vi "Load-GUI-values-from-file.vi"(8 "error in":errorcluster, 10 "UI ref. in":refnum<data-value>, 11 "Data ref. in":refnum<data-value>) -> (0 "error IO":errorcluster, 2 "UI ref.":refnum<data-value>, 3 "Data ref.":refnum<data-value>)   [LabVIEW 2013, in "CameraVision.lvlib" / "CV-Main.lvclass"]
doc: "This function loads and overwrites new values for the GUI parameters. The values are obtained from an .xml settings file. The user is warned that the parameters will be overwritten and has the possibility to cancel the operation.\nDepending on the 'Settings source' GUI control, 4 cases are possible:\n- 'Custom': the 'Load settings' button is disabled, no action is taken.\n- 'Default': the default values of the GUI parameters are loaded from '<Application>\\Program data\\parameters-gui.xml'.\n- 'Last used': the last succesfully used vales are loaded (can be from previous program execution) from '<Application>\\Program data\\last.xml'.\n- 'Saved': the user is prompted to choose an .xml file through a standard file browser window. If the selected file is not valid, an error message is displayed."
uses:
  CV-Main.lvclass
  UI/CV-UI.lvclass
  UI/Popup-messages.ctl
  UI/CV-UI.lvclass/CV-UI.ctl
  UI/Read Settings-source.vi
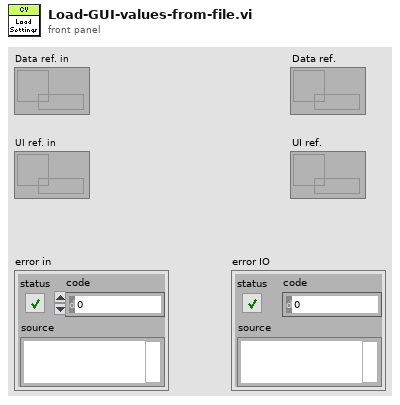
[diagram p1: front panel]
types:
  T1 = typedef "CameraVision.lvlib/CV-UI.lvclass/Popup-messages.ctl" = enum16{"Error-Black image", "Error-Camera config file", "Error-Camera connect", "Error-Grabber init", "Error-Camera setting", "Error-Image offset", "Error-Image import", "Error-Settings file not exist", "Error-Timing source", "Conflict-Filters", "Conflict-Map", "Conflict-Framerate", "Conflict-Charact", "Conflict-Temperature field", "Conflict-Temperature value", "Conflict-Storage-Binary image", "Conflict-Storage-Corrected image", "Conflict-Storage-Map", "Conflict-Storage-Charact", "Conflict-Storage-Temperature field", "Conflict-Storage-Temperature value", "Warning-File exist", "Warning-Parameter reset", "Warning-User cancel", "Info-Images imported"}
  T2 = typedef "CameraVision.lvlib/CV-UI.lvclass/Settings-source.ctl" = enum16{"Custom", "Default", "Last used", "File"}
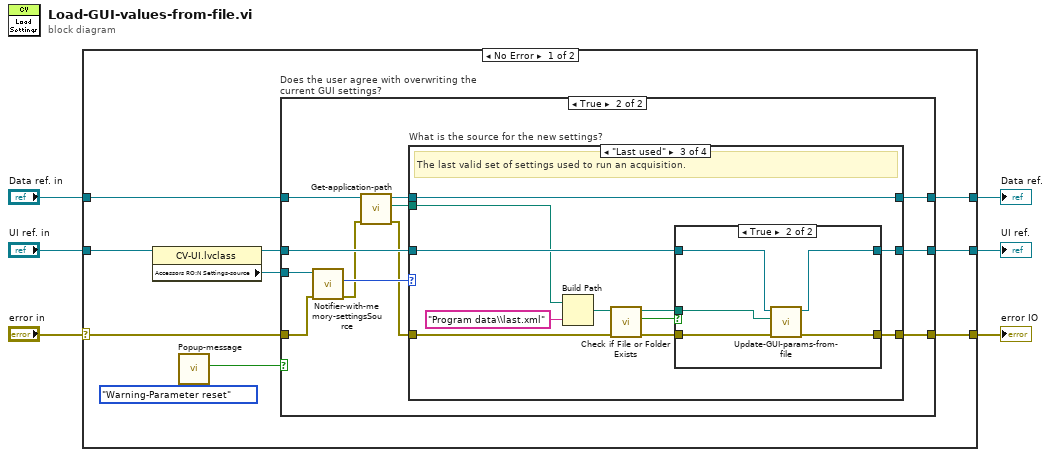
[diagram p0: block diagram]
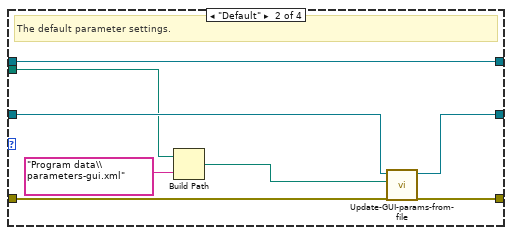
[diagram p4: hidden frame]
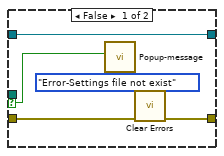
[diagram p5: hidden frame]
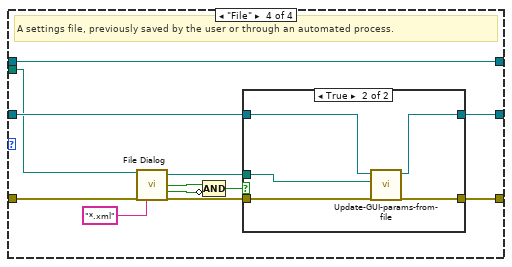
[diagram p6: hidden frame]
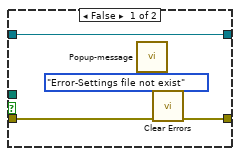
[diagram p7: hidden frame]
diagram:
  n1 = case shown="No Error" "error in" {
    selector: "error in" -> [w15 w87]
    tunnel: [w16 w87] -> w6
    tunnel: "UI ref. in" -> [w14 w86]
    tunnel: [w11 w86] -> w3
    tunnel: "Data ref. in" -> [w10 w85]
    tunnel: [w9 w85] -> w1
    frame No Error {
      n2 = property class="CV-UI.lvclass"(reference=w14) -> (reference out=w12:refnum<data-value>, "Accessors RO:N Settings-source"=w13:refnum<notifier>)  [unwired: 1 in, 1 out]
      n3 = call "Popup-message.vi"("Message"=Popup-messages."Warning-Parameter reset") -> ("Return"=w8:bool)  [unwired: 10 in]
      n4 = case "Does the user agree with overwriting the current GUI settings?" shown="True" w8 {
        tunnel: [w19 w31] -> w16
        tunnel: w15 -> [w19 w28]
        tunnel: w13 -> [_ w30]
        tunnel: w12 -> [w18 w27]
        tunnel: [w18 w26] -> w11
        tunnel: w10 -> [w17 w25]
        tunnel: [w17 w20] -> w9
        frame False {
        }
        frame True {
          n5 = call "Notifier-with-memory-settingsSource.vi"("error in"=w28, "Notifier in"=w30) -> ("error IO"=w24:errorcluster, "Notification"=w29:T2)  [unwired: 8 in]
          n6 = call "Get-application-path.vi"("error in (no error)"=w24, "Data ref. in"=w25) -> ("error out"=w23:errorcluster, "App path"=w22:path, "Data ref."=w21:refnum<data-value>)  [unwired: 7 in]
          n7 = case "What is the source for the new settings?" shown="\"Last used\"" w29 {
            tunnel: [w34 w42 w49 w75] -> w31
            tunnel: w23 -> [w34 w41 w51 w67]
            tunnel: w27 -> [w33 w38 w46 w68]
            tunnel: [w33 w37 w45 w66] -> w26
            tunnel: w22 -> [_ w36 w44 w65]
            tunnel: w21 -> [w32 w35 w43 w64]
            tunnel: [w32 w35 w43 w64] -> w20
            frame "Custom", Default {
              # "A cutom set of settings, as currently visible on the graphical user interface."
            }
            frame "Default" {
              # "The default parameter settings."
              n8 = Build Path(base path=w36, name or relative path="Program data\\parameters-gui.xml" ("Relative save path")) -> (appended path=w39:path)
              n9 = call "Update-GUI-params-from-file.vi"("error in"=w41, "File path"=w39, "UI ref. in"=w38) -> ("error IO"=w42:errorcluster, "UI ref."=w37:refnum<data-value>)  [unwired: 7 in]
            }
            frame "Last used" {
              # "The last valid set of settings used to run an acquisition."
              n10 = Build Path(base path=w44, name or relative path="Program data\\last.xml" ("string")) -> (appended path=w52:path)
              n11 = call <vilib>:"Check if File or Folder Exists.vi"("error in (no error)"=w51, "path"=w52) -> ("error out"=w50:errorcluster, "file or folder exists?"=w47:bool, "dup path"=w48:path)  [unwired: 7 in]
              n12 = case shown="True" w47 {
                selector: w47 -> [w56 _]
                tunnel: w50 -> [w58 w63]
                tunnel: [w54 w62] -> w49
                tunnel: w48 -> [_ w61]
                tunnel: w46 -> [w57 w60]
                tunnel: [w57 w59] -> w45
                frame False {
                  n13 = call "Popup-message.vi"("Message"=Popup-messages."Error-Settings file not exist", "Ignore?"=w56) -> ()  [unwired: 9 in, 1 out]
                  n14 = call <vilib>:"Clear Errors.vi"("error in (no error)"=w58) -> ("error out"=w54:errorcluster)  [unwired: 6 in]
                }
                frame True {
                  n15 = call "Update-GUI-params-from-file.vi"("error in"=w63, "File path"=w61, "UI ref. in"=w60) -> ("error IO"=w62:errorcluster, "UI ref."=w59:refnum<data-value>)  [unwired: 7 in]
                }
              }
            }
            frame "File" {
              # "A settings file, previously saved by the user or through an automated process."
              n16 = call "File Dialog"("start path"=w65, "error in"=w67, "pattern (all files)"="*.xml") -> ("selected path"=w72:path, "exists"=w71:bool, "cancelled"=w70:bool, "error out"=w73:errorcluster)  [unwired: 9 in]
              n17 = Compound Arithmetic op=AND(w71, invert w70) -> (w69:bool)
              n18 = case shown="True" w69 {
                tunnel: w73 -> [w79 w84]
                tunnel: [w78 w83] -> w75
                tunnel: w72 -> [_ w81]
                tunnel: w68 -> [w77 w82]
                tunnel: [w77 w80] -> w66
                frame False {
                  n19 = call "Popup-message.vi"("Message"=Popup-messages."Error-Settings file not exist") -> ()  [unwired: 10 in, 1 out]
                  n20 = call <vilib>:"Clear Errors.vi"("error in (no error)"=w79) -> ("error out"=w78:errorcluster)  [unwired: 6 in]
                }
                frame True {
                  n21 = call "Update-GUI-params-from-file.vi"("error in"=w84, "File path"=w81, "UI ref. in"=w82) -> ("error IO"=w83:errorcluster, "UI ref."=w80:refnum<data-value>)  [unwired: 7 in]
                }
              }
            }
          }
        }
      }
    }
    frame Error {
    }
  }
  "error IO" <- w6
  "UI ref." <- w3
  "Data ref." <- w1
